vi "PulseOxControl.vi"() -> ()   [LabVIEW 2016]
uses:
  <vilib>/Instr/_visa.llb/VISA Configure Serial Port (Instr).vi
panel:
  in  "PILOT_PA [7..0]":u8=127 format="%x"
  in  "OK Button 3":bool
  in  "LED2_PA [7..0]":u8=36 format="%x"
  in  "OK Button 2":bool
  in  "OK Button":bool
  in  "LED1_PA [7..0]":u8=36 format="%x"
  out "DEVICE OK":bool
  in  "COM Select":refnum<visa-resource-name>="COM3"
  out "O2 SAT":dbl
  out "PULSE":dbl
  in  "Upper Cut-Off":dbl=75.0
  in  "Lower Cut-Off":dbl=10.0
  out "Sphygmogram":dynamicdata(graph)
  in  "Array 2":dbl[](array[numeric])=array[6515 elements]
  in  "Array":dbl[](array[numeric])=array[6516 elements]
  in  "STOP":bool
  # "Filter Settings"
  # "LED Current Control"
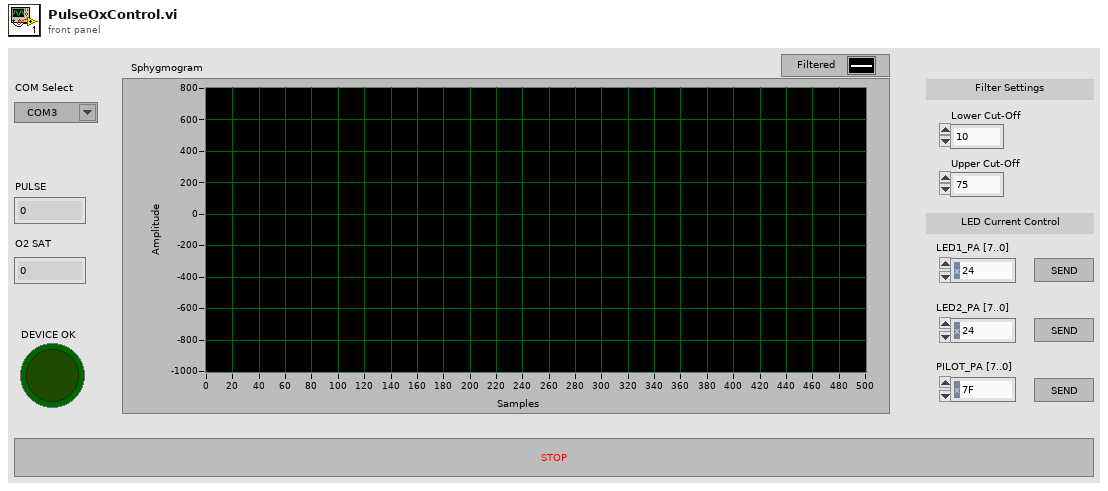
[diagram p1: front panel]
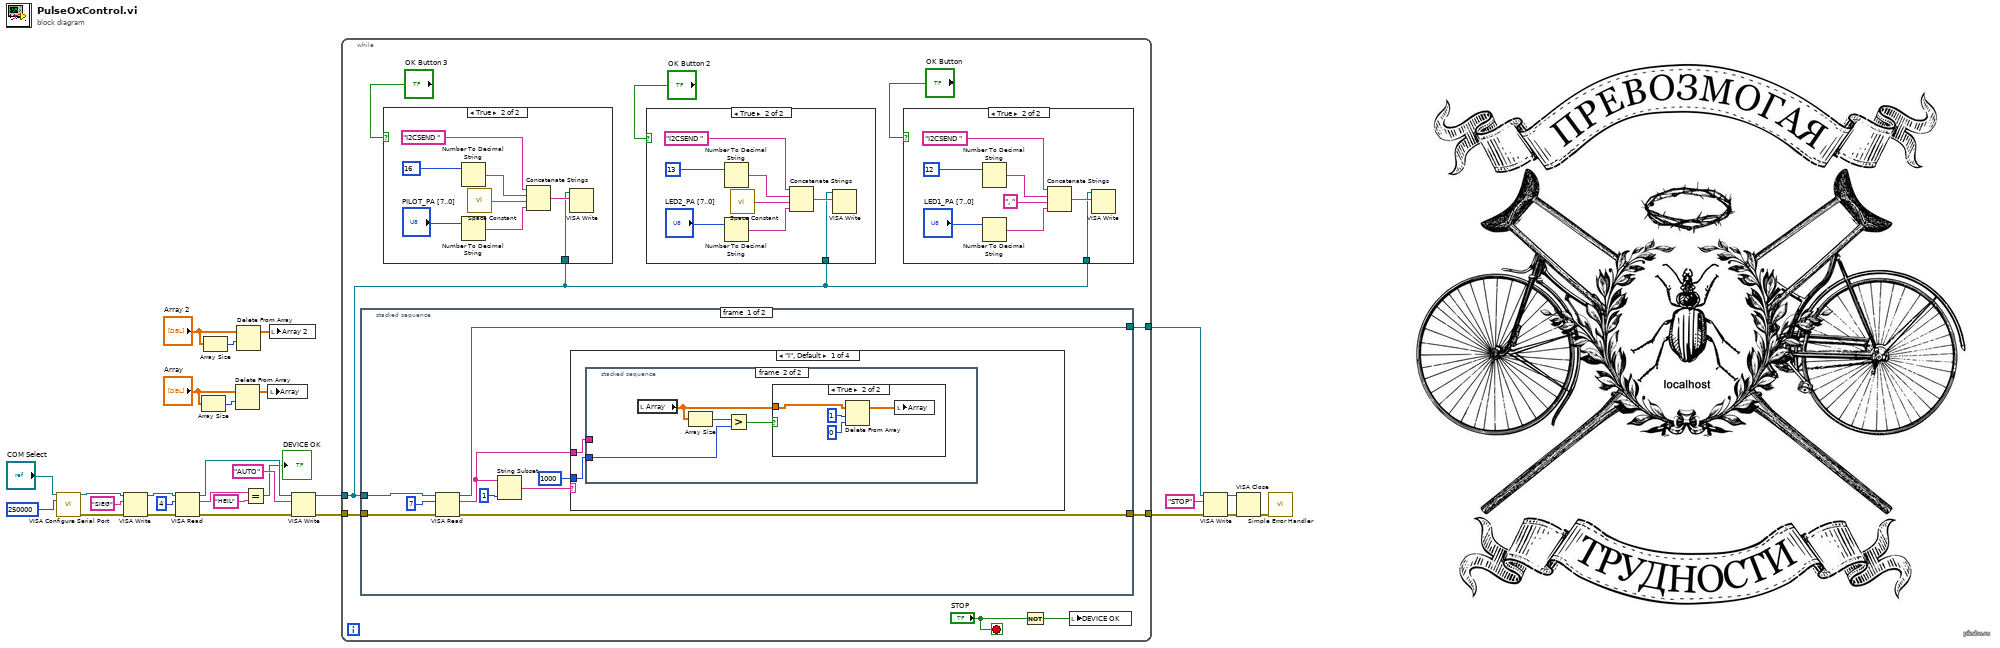
[diagram p0: block diagram]
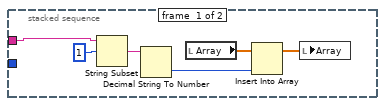
[diagram p5: hidden frame]
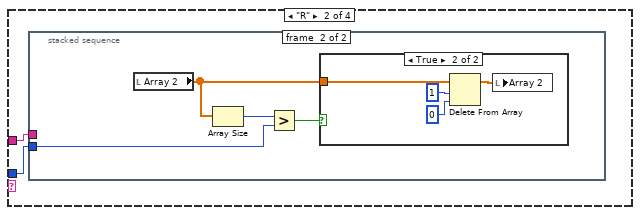
[diagram p7: hidden frame]
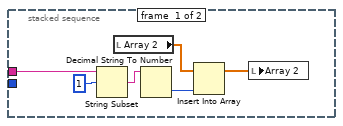
[diagram p8: hidden frame]
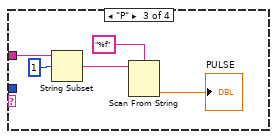
[diagram p10: hidden frame]
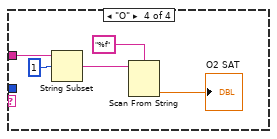
[diagram p11: hidden frame]
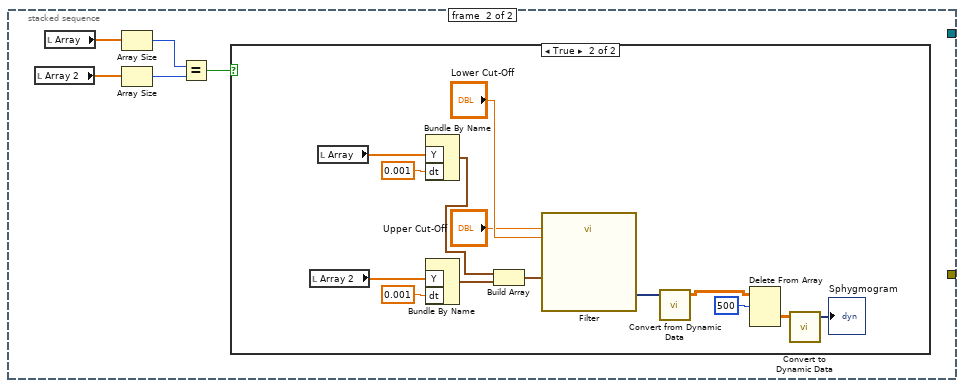
[diagram p12: hidden frame]
diagram:
  n1 = call-poly "VISA Configure Serial Port"("VISA resource name"="COM Select", "baud rate (9600)"=u32 250000) -> ("VISA resource name out"=w16:refnum<visa-resource-name>, "error out"=w15:errorcluster)  [unwired: 12 in]
  n2 = VISA Write(VISA resource name=w16, write buffer="SIEG", error in (no error)=w15) -> (VISA resource name out=w12:refnum<visa-resource-name>, error out=w11:errorcluster)  [unwired: 1 out]
  n3 = VISA Read(VISA resource name=w12, byte count=u32 4, error in (no error)=w11) -> (VISA resource name out=w9:refnum<visa-resource-name>, read buffer=w8:string, error out=w10:errorcluster)  [unwired: 1 out]
  n4 = Array Size(array="Array") -> (size(s)=w19:i32)
  n5 = Array Size(array="Array 2") -> (size(s)=w21:i32)
  n6 = Delete From Array(array="Array", length=w19) -> (array with subset deleted=w24:dbl[])  [unwired: 1 in, 1 out]
  n7 = Delete From Array(array="Array 2", length=w21) -> (array with subset deleted=w23:dbl[])  [unwired: 1 in, 1 out]
  n8 = Equal?(x=w8, y="HEIL") -> (x = y?=→"DEVICE OK":bool)
  n9 = local write "Array"(w24) -> ()
  n10 = local write "Array 2"(w23) -> ()
  n11 = VISA Write(VISA resource name=w9, write buffer="AUTO", error in (no error)=w10) -> (VISA resource name out=w27:refnum<visa-resource-name>, error out=w26:errorcluster)  [unwired: 1 out]
  n12 = while {
    tunnel: [w37] -> w3
    tunnel: w27 -> [w29]
    tunnel: w26 -> [w36]
    tunnel: [w35] -> w2
    stop <- "STOP" stop-if-true
    n13 = stacked-sequence {
      tunnel: [w62 _] -> w37
      tunnel: w29 -> [w69 _]
      tunnel: w36 -> [w66 _]
      tunnel: [w63 _] -> w35
      frame #0 {
        n14 = VISA Read(VISA resource name=w69, byte count=u32 7, error in (no error)=w66) -> (VISA resource name out=w62:refnum<visa-resource-name>, read buffer=w65:string, error out=w63:errorcluster)  [unwired: 1 out]
        n15 = String Subset(string=w65, length (rest)=1 ("length (rest)")) -> (substring=w67:string)  [unwired: 1 in]
        n16 = case shown="\"I\", Default" w67 {
          tunnel: w65 -> [w72 w88 w106 w111]
          tunnel: 1000 ("y") -> [w71 w87 _ _]
          frame "I", Default {
            n17 = stacked-sequence {
              tunnel: w72 -> [w77 _]
              tunnel: w71 -> [_ w81]
              frame #0 {
                n18 = String Subset(string=w77, offset (0)=1) -> (substring=w76:string)  [unwired: 1 in]
                n19 = Decimal String To Number(string=w76) -> (number=w74:i32)  [unwired: 2 in, 1 out]
                n20 = local read "Array"() -> (w75:dbl[])
                n21 = Insert Into Array(array=w75, new element=w74) -> (w73:dbl[])  [unwired: 1 in]
                n22 = local write "Array"(w73) -> ()
              }
              frame #1 {
                n23 = local read "Array"() -> (w79:dbl[])
                n24 = Array Size(array=w79) -> (size(s)=w82:i32)
                n25 = Greater?(x=w82, y=w81) -> (0:w80:bool)
                n26 = case shown="True" w80 {
                  tunnel: w79 -> [_ w86]
                  frame False {
                  }
                  frame True {
                    n27 = Delete From Array(array=w86, length=1, index=0) -> (array with subset deleted=w83:dbl[])  [unwired: 1 out]
                    n28 = local write "Array"(w83) -> ()
                  }
                }
              }
            }
          }
          frame "R" {
            n29 = stacked-sequence {
              tunnel: w88 -> [w94 _]
              tunnel: w87 -> [_ w95]
              frame #0 {
                n30 = String Subset(string=w94, offset (0)=1) -> (substring=w92:string)  [unwired: 1 in]
                n31 = local read "Array 2"() -> (w91:dbl[])
                n32 = Decimal String To Number(string=w92) -> (number=w90:i32)  [unwired: 2 in, 1 out]
                n33 = Insert Into Array(array=w91, new element=w90) -> (w89:dbl[])  [unwired: 1 in]
                n34 = local write "Array 2"(w89) -> ()
              }
              frame #1 {
                n35 = local read "Array 2"() -> (w96:dbl[])
                n36 = Array Size(array=w96) -> (size(s)=w98:i32)
                n37 = Greater?(x=w98, y=w95) -> (0:w97:bool)
                n38 = case shown="True" w97 {
                  tunnel: w96 -> [_ w102]
                  frame False {
                  }
                  frame True {
                    n39 = Delete From Array(array=w102, length=1, index=0) -> (array with subset deleted=w99:dbl[])  [unwired: 1 out]
                    n40 = local write "Array 2"(w99) -> ()
                  }
                }
              }
            }
          }
          frame "P" {
            n41 = String Subset(string=w106, offset (0)=1) -> (substring=w104:string)  [unwired: 1 in]
            n42 = Scan From String(format string="%f", input string=w104) -> (output 1=→"PULSE":dbl)  [unwired: 3 in, 3 out]
          }
          frame "O" {
            n43 = String Subset(string=w111, offset (0)=1) -> (substring=w108:string)  [unwired: 1 in]
            n44 = Scan From String(format string="%f", input string=w108) -> (output 1=→"O2 SAT":dbl)  [unwired: 3 in, 3 out]
          }
        }
      }
      frame #1 {
        n45 = local read "Array 2"() -> (w117:dbl[])
        n46 = local read "Array"() -> (w116:dbl[])
        n47 = Array Size(array=w116) -> (size(s)=w115:i32)
        n48 = Array Size(array=w117) -> (size(s)=w114:i32)
        n49 = Equal?(x=w115, y=w114) -> (x = y?=w113:bool)
        n50 = case shown="True" w113 {
          frame False {
          }
          frame True {
            n51 = local read "Array 2"() -> (w130:dbl[])
            n52 = local read "Array"() -> (w131:dbl[])
            n53 = Bundle By Name("Y"=w131, "dt"=0.001) -> (w126:waveform(dbl))  [unwired: 1 in]
            n54 = Bundle By Name("Y"=w130, "dt"=0.001) -> (w127:waveform(dbl))  [unwired: 1 in]
            n55 = Build Array(w126, w127) -> (w121:waveform(dbl)[])
            n56 = call "Filter"("Lower Cut-Off"="Lower Cut-Off", "Upper Cut-Off"="Upper Cut-Off", "Signal"=w121) -> ("Filtered Signal"=w120:dynamicdata)  [unwired: 7 in, 1 out]
            n57 = call "Convert from Dynamic Data"("Dynamic Data Type"=w120) -> ("Array"=w124:dbl[][])  [unwired: 3 in]
            n58 = Delete From Array(array=w124, length=500) -> (deleted portion=w119:dbl[][])  [unwired: 2 in, 1 out]
            n59 = call "Convert to Dynamic Data"("2D Array"=w119) -> ("Dynamic Data Type"=→"Sphygmogram":dynamicdata)  [unwired: 3 in]
          }
        }
      }
    }
    n60 = case shown="True" "OK Button 3" {
      tunnel: w29 -> [_ w38]
      frame False {
      }
      frame True {
        n61 = Number To Decimal String(number=u8 16) -> (decimal integer string=w40:string)  [unwired: 1 in]
        n62 = Number To Decimal String(number="PILOT_PA [7..0]") -> (decimal integer string=w42:string)  [unwired: 1 in]
        n63 = call <vilib>:"Space Constant.vi"() -> ("String"=w43:string)
        n64 = Concatenate Strings("I2CSEND ", w40, w43, w42) -> (w39:string)
        n65 = VISA Write(VISA resource name=w38, write buffer=w39) -> ()  [unwired: 1 in, 3 out]
      }
    }
    n66 = case shown="True" "OK Button 2" {
      tunnel: w29 -> [_ w46]
      frame False {
      }
      frame True {
        n67 = Number To Decimal String(number=u8 13) -> (decimal integer string=w48:string)  [unwired: 1 in]
        n68 = Number To Decimal String(number="LED2_PA [7..0]") -> (decimal integer string=w50:string)  [unwired: 1 in]
        n69 = call <vilib>:"Space Constant.vi"() -> ("String"=w51:string)
        n70 = Concatenate Strings("I2CSEND ", w48, w51, w50) -> (w47:string)
        n71 = VISA Write(VISA resource name=w46, write buffer=w47) -> ()  [unwired: 1 in, 3 out]
      }
    }
    n72 = case shown="True" "OK Button" {
      tunnel: w29 -> [_ w55]
      frame False {
      }
      frame True {
        n73 = Number To Decimal String(number=u8 12) -> (decimal integer string=w57:string)  [unwired: 1 in]
        n74 = Number To Decimal String(number="LED1_PA [7..0]") -> (decimal integer string=w59:string)  [unwired: 1 in]
        n75 = Concatenate Strings("I2CSEND ", w57, ", ", w59) -> (w56:string)
        n76 = VISA Write(VISA resource name=w55, write buffer=w56) -> ()  [unwired: 1 in, 3 out]
      }
    }
    n77 = Not(x="STOP") -> (.not. x?=w34:bool)
    n78 = local write "DEVICE OK"(w34) -> ()
  }
  n79 = VISA Write(VISA resource name=w3, write buffer="STOP", error in (no error)=w2) -> (VISA resource name out=w4:refnum<visa-resource-name>, error out=w5:errorcluster)  [unwired: 1 out]
  n80 = VISA Close(VISA resource name=w4, error in (no error)=w5) -> (error out=w28:errorcluster)
  n81 = call <vilib>:"Simple Error Handler.vi"("error in (no error)"=w28) -> ()  [unwired: 4 in, 5 out]
